vi "Thermometer.vi"() -> ()   [LabVIEW 2010]
panel:
  out "String":string
  in  "Unit":bool
  out "Celsius":dbl
  out "Thermometer":dbl(slide) scale=0.0..100.0
  out "Temp. in C":dbl
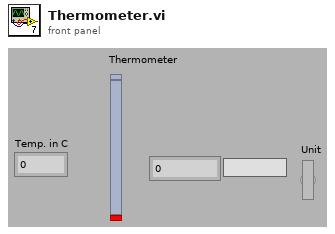
[diagram p1: front panel]
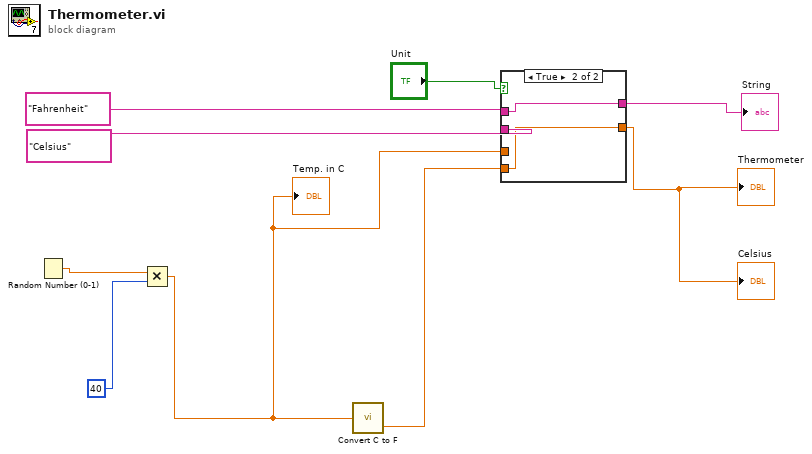
[diagram p0: block diagram]
diagram:
  n1 = Random Number (0-1)() -> (number: 0 to 1=w9:dbl)
  n2 = Multiply(x=w9, y=40) -> (x*y=w7:dbl)
  "Temp. in C" <- w7
  n3 = call "Convert C to F.vi"("Temp in C"=w7) -> ("Temp in F"=w6:dbl)  [unwired: 1 in]
  n4 = case shown="True" "Unit" {
    tunnel: w7 -> [w11 _]
    tunnel: w6 -> [_ w13]
    tunnel: [w11 w13] -> w4
    tunnel: "Celsius" -> [w10 _]
    tunnel: "Fahrenheit" -> [_ w12]
    tunnel: [w10 w12] -> w1
    frame False {
    }
    frame True {
    }
  }
  "Thermometer" <- w4
  "Celsius" <- w4
  "String" <- w1
